vi "GetRectangle__slk_mt.vi"(8 "error in (no error)":errorcluster, 11 "segment in":refnum<class "Segment__slk_mt.lvclass">) -> (0 "error out":errorcluster, 2 "rectangle":T1, 3 "segment out":refnum<class "Segment__slk_mt.lvclass">)   [LabVIEW 2015, in "Lazyboots Menu Tool.lvlib" / "Segment__slk_mt.lvclass"]
doc: "Returns rectangle of the segment."
uses:
  <vilib>/SLK/Lazyboots Menu Tool/Private/AddLabel/Class/Segment/Segment__slk_mt.lvclass
  <vilib>/SLK/Lazyboots Menu Tool/Private/AddLabel/Class/Segment/Segment__slk_mt.lvclass/Segment__slk_mt.ctl
panel:
  # "GetRectangle__slk_mt.vi\nReturns rectangle of the segment.\n\nNOTICE -- YOU MUST LEAVE THIS NOTICE IN PLACE.\n\nCopyright (c) 2011, LIANG LIU Shawn.Liu.cn@gmail.com\nAll rights reserved.\n\nRedistribution and use in source and binary forms, with or without modification, are permitted provided that the following conditions are met:\n-Redistributions of source code must retain the above copyright notice, this list of conditions and the following disclaimer.\n-Redistributions in binary form must reproduce the above copyright notice, this list of conditions and the following disclaimer in the documentation and/or other materials provided with the distribution.\n-Neither the name of the eLp nor the names of its contributors may be used to endorse or promote products derived from this software without specific prior written permission.\n\nTHIS SOFTWARE IS PROVIDED BY THE COPYRIGHT HOLDERS AND CONTRIBUTORS \"AS IS\" AND ANY EXPRESS OR IMPLIED WARRANTIES, INCLUDING, BUT NOT LIMITED TO, THE IMPLIED WARRANTIES OF MERCHANTABILITY AND FITNESS FOR A PARTICULAR PURPOSE ARE DISCLAIMED. IN NO EVENT SHALL THE COPYRIGHT HOLDER OR CONTRIBUTORS BE LIABLE FOR ANY DIRECT, INDIRECT, INCIDENTAL, SPECIAL, EXEMPLARY, OR CONSEQUENTIAL DAMAGES (INCLUDING, BUT NOT LIMITED TO, PROCUREMENT OF SUBSTITUTE GOODS OR SERVICES; LOSS OF USE, DATA, OR PROFITS; OR BUSINESS INTERRUPTION) HOWEVER CAUSED AND ON ANY THEORY OF LIABILITY, WHETHER IN CONTRACT, STRICT LIABILITY, OR TORT (INCLUDING NEGLIGENCE OR OTHERWISE) ARISING IN ANY WAY OUT OF THE USE OF THIS SOFTWARE, EVEN IF ADVISED OF THE POSSIBILITY OF SUCH DAMAGE."
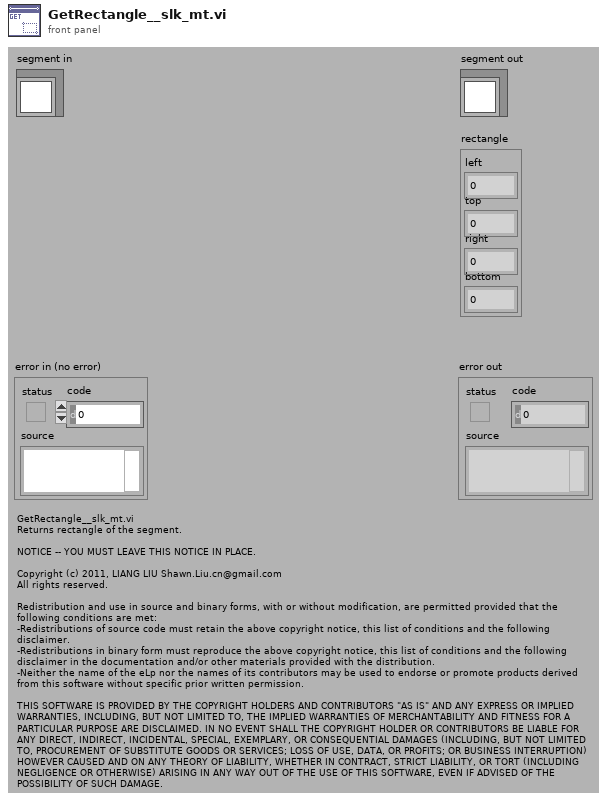
[diagram p1: front panel]
types:
  T1 = cluster{"left":i16, "top":i16, "right":i16, "bottom":i16}
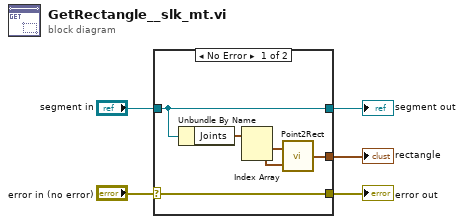
[diagram p0: block diagram]
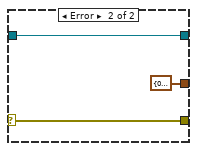
[diagram p2: hidden frame]
diagram:
  n1 = case shown="No Error" "error in (no error)" {
    selector: "error in (no error)" -> [w11 w14]
    tunnel: [w11 w14] -> w4
    tunnel: [w10 w13] -> w2
    tunnel: "segment in" -> [w10 w13]
    tunnel: [w6 T1 {"left"=0, "top"=0, "right"=0, "bottom"=0} ("rect")] -> w1
    frame No Error {
      n2 = Unbundle By Name(w10) -> ("Joints"=w9:cluster{"X":i32, "Y":i32}[])
      n3 = Index Array(array=w9) -> (element #1=w8:cluster{"X":i32, "Y":i32}, element #2=w7:cluster{"X":i32, "Y":i32})  [unwired: 2 in]
      n4 = call <vilib>:"Point2Rect.vi"("point b"=w7, "point a"=w8) -> ("rect"=w6:T1)
    }
    frame Error {
    }
  }
  "error out" <- w4
  "segment out" <- w2
  "rectangle" <- w1
